vi "FileNaming.vi"(7 "Clock":timestamp, 9 "File Name Out":string, 10 "File Format":string, 11 "Data Collection Folder":path) -> (3 "path":path)   [LabVIEW 2022 SP3]
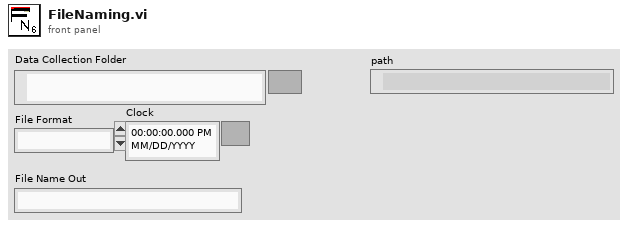
[diagram p1: front panel]
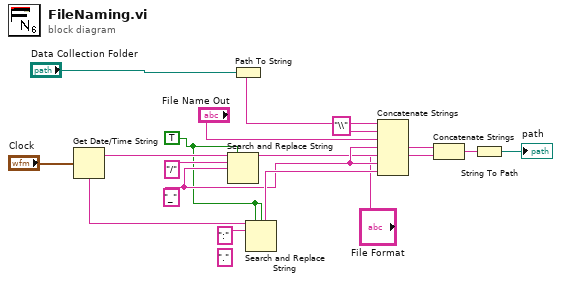
[diagram p0: block diagram]
diagram:
  w4 = TRUE ("replace all? (F)")
  (unwired) "." ("replace string (\"\")")
  w14 = "_" ("string")
  n1 = Get Date/Time String(seconds (now)="Clock") -> (date string=w9:string, time string=w12:string)  [unwired: 2 in]
  n2 = Search and Replace String(replace all?=w4, input string=w9, search string="/", replace string=w14) -> (result string=w11:string)  [unwired: 4 in, 3 out]
  n3 = Path To String(path="Data Collection Folder") -> (string=w6:string)
  n4 = Search and Replace String(replace all?=w4, case sensitive?=w4, input string=w12, search string=":") -> (result string=w15:string)  [unwired: 4 in, 3 out]
  n5 = Concatenate Strings(w6, "\\" ("string"), "File Name Out", w14, w11, w14, w15) -> (w16:string)
  n6 = Concatenate Strings(w16, "File Format") -> (w17:string)
  n7 = String To Path(string=w17) -> (path=→"path":path)
